vi "Error_Log_Init.vi"(6 "Error Log Folder Name":string, 7 "Configuration File's Section Name":string, 9 "Configuration File Name":string, 10 "Configuration File's Folder and Error Log's Folder":i32, 11 "Application Name (Application)":string) -> (0 "error out":errorcluster)   [LabVIEW 2011]
uses:
  <userlib>/_JGCODE/error_logger/_error_logger.llb/ErrorLogger.lvclass
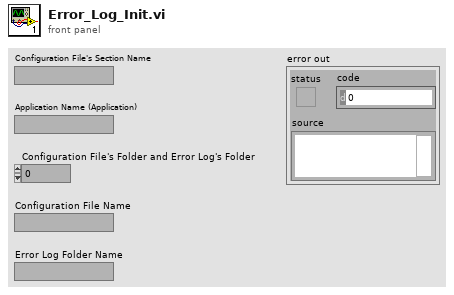
[diagram p1: front panel]
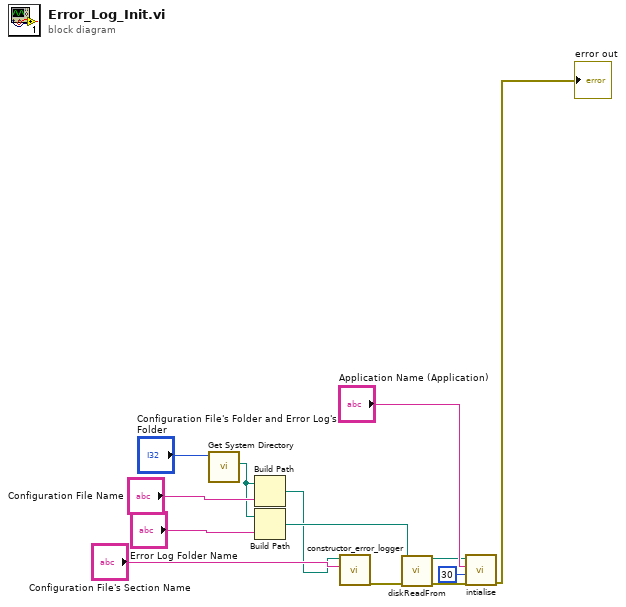
[diagram p0: block diagram]
diagram:
  n1 = call <vilib>:"Get System Directory.vi"("system directory type"="Configuration File's Folder and Error Log's Folder") -> ("system directory"=w3:path)  [unwired: 10 in]
  n2 = Build Path(base path=w3, name or relative path="Configuration File Name") -> (appended path=w5:path)
  n3 = Build Path(base path=w3, name or relative path="Error Log Folder Name") -> (appended path=w8:path)
  n4 = call <userlib>:"constructor_error_logger.vi"("File Section"="Configuration File's Section Name", "File Path"=w5) -> ("error out"=w7:errorcluster)  [unwired: 9 in]
  n5 = call <userlib>:"diskReadFrom.vi"("error in (no error)"=w7) -> ("error out"=w9:errorcluster)  [unwired: 10 in]
  n6 = call <userlib>:"intialise.vi"("error in (no error)"=w9, "Maximum Number Of Files (30)"=30, "Application Name (Application)"="Application Name (Application)", "Error Log Folder"=w8) -> ("error out"=→"error out":errorcluster)  [unwired: 6 in, 1 out]
